vi "Master Setup File Fault Check.vi"(0 "Reset?":bool, 5 "Clear File Load Error Ref.":refnum<vi>, 7 "Pattern Label":T2 items=["Channel Setup (0)", "PID Setup (1)", "Filter Setup (2)", "~Reserved Old CAN Msgs (3)", "~Reserved Old CAN1 (4)", "~Reserved Old CAN2 (5)", "Digital Inputs Setup (6)", "Digital Outputs Setup (7)", "Logging 1 Setup (8)", "Logging 2 Setup (9)", "Logging 3 Setup (10)", "Setpoint Setup (11)", "Test Series Setup (12)", "Graph Setup (13)", "System Configure (14)", "Header (15)", "Profile Manager (16)", "Post-Mortem Logging (17)", "High-Speed Data (18)", "Statistic Channel Setup (19)", "Ramp Channel Setup (20)", "ETAS INCA Channel Setup (21)", "ETC ECCS Transducer Setup (22)", "ETC ECCS Test Setup (23)", "AVL AK Smoke Meter Setup (24)", "Triggers Setup (25)", "Alarm Limits Setup (26)", "YKWT1 Measurement (27)", "YKWT1 Instrument (28)", "Auto File Settings (29)", "Playback File Setting (30)", "UUT Constants (31)", "UPS Setup (32)", "Differential Channel Setup (33)", "Integral Channel Setup (34)", "Signal Channel Setup (35)", "Calibration Setup (36)", "BNC Setup (37)", "ASAP3 Setup (38)", "Chassis Force Calculations (39)", "Chassis Teststand Losses (40)", "Chassis Vehicle Losses (41)", "Formula Channels (42)", "ASAP3 Map Coords Setup (43)", "Digital Controls Setup (44)", "Push Buttons Setup (45)", "Sliders Setup (46)", "~Reserved~ (47)", "Email Setup (48)", "Timer Setup (49)", "Unit Conversion Setup (50)", "Visible Channels (51)", "Main Display Setup (52)", "Message Display Setup (53)", "Input Display Setup (54)", "Unico Parameter Downloads (55)", "Flow Meter Setup (56)", "Channel Zero Offset (57)", "YKWT2 Measurement (58)", "YKWT2 Instrument (59)", "~Reserved Old CAN3 (60)", "CAS Setup (61)", "Accumulation Channel Setup (62)", "Valvetrain Dynamics Setup (63)", "CCP Setup (64)", "System Log Setup (65)", "Throttle Controller (66)", "RE Shifter (67)", "Main Display (68)", "~Reserved~ (69)", "FlexRay (70)", "YKWT3 Measurement (71)", "YKWT3 Instrument (72)", "CAN XNET API (73)"], 9 "File Operation":T1, 11 "error in (no error)":errorcluster) -> (4 "Module Fault Array":bool[](array[boolean]), 15 "error out":errorcluster)   [LabVIEW 2017]
uses:
  Master Setup Pattern Enum.ctl
  Setup File Operations/File Operation with History.ctl
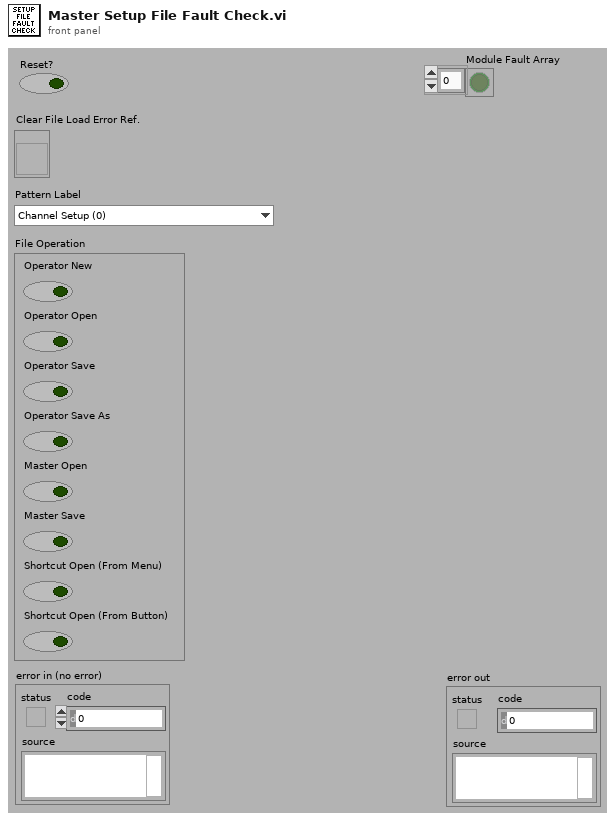
[diagram p1: front panel]
types:
  T1 = typedef "File Operation with History.ctl" = cluster{"Operator New":bool, "Operator Open":bool, "Operator Save":bool, "Operator Save As":bool, "Master Open":bool, "Master Save":bool, "Shortcut Open (From Menu)":bool, "Shortcut Open (From Button)":bool}
  T2 = typedef "Master Setup Pattern Enum.ctl" = i32
  T3 = typedef "PC_INI_Data__TypeDef.ctl" = cluster{"REPS Version":T4, "System Configuration":T5, "OPC PLC Write":string, "OPC PLC Read":string, "Modbus Info":string, "INCA Configuration":cluster{"IP":string, "Port":i32, "Protocol Version":i32}, "ECCS Setup":cluster{"Enable":bool, "IP":string, "TCP Port":u16, "UDP Port":u16, "Engine ODBC Name":string, "Fuel ODBC Name":string}, "Encoder Configuration":cluster{"Encoder1PPR":i32, "Encoder1Interval1":i32, "Encoder1Interval2":i32, "Roll Diameter(Feet)":i32, "Encoder2PPR":i32, "Encoder3PPR":i32, "Encoder4PPR":i32, "Encoder5PPR":i32, "Encoder2Interval1":i32, "Encoder2Interval2":i32, "Encoder3Interval1":i32, "Encoder3Interval2":i32}, "Pickup1 Configuration":cluster{"PickupPPR":i32, "PickupInterval1":i32, "PickupInterval2":i32}, "Pickup2 Configuration":cluster{"PickupPPR":i32, "PickupInterval1":i32, "PickupInterval2":i32}, "Pickup3 Configuration":cluster{"PickupPPR":i32, "PickupInterval1":i32, "PickupInterval2":i32}, "Shifter Configuration":cluster{"RE Shifter Enable":bool, "Shifter IP Address":string, "Shifter Port":u16}, "Misc Configuration":T6, "Logging Configuration":cluster{"Number of Log Channels":dbl, "Max Log  File Size":dbl}}
  T4 = typedef "REPS Version.ctl" = cluster{"Version":string}
  T5 = typedef "System Configuration.ctl" = cluster{"Cell":string, "DualMotorSet":bool, "Hardware Setup Array":bool[], "Host IP":string, "Remote IP 1":string, "Remote IP 2":string, "Remote IP 3":string, "Remote Enable 1":bool, "Remote Enable 2":bool, "Remote Enable 3":bool, "Company Name":string, "Company Info":string, "Number Of Modbus":i32, "Setup Files Path":path, "Master File Path":path, "Master Setup Titles":string[], "Encoder1PPR":i32, "Encoder1Interval1":i32, "Encoder1Interval2":i32, "Display File Error Status?":bool[], "Update to RT Delay":u32, "Formula Rate (Hz)":u32, "Custom Screen (Left) Path":path, "Custom Screen (Right) Path":path}
  T6 = typedef "Misc Configuration.ctl" = cluster{"Show PM Logging Indicator":bool}
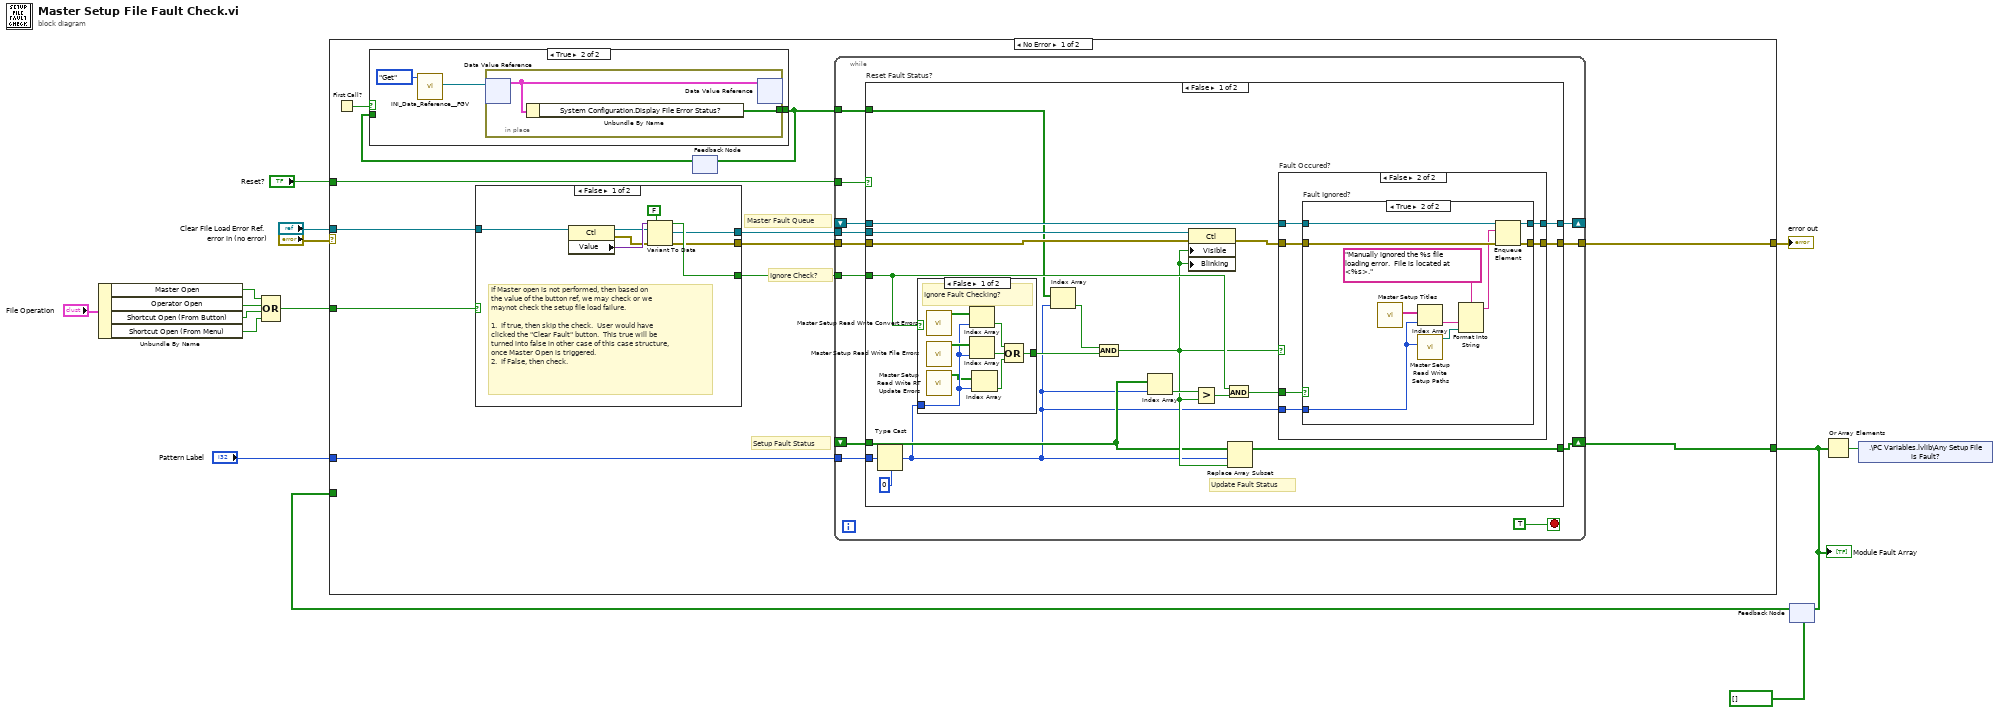
[diagram p0: block diagram]
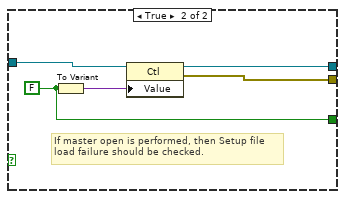
[diagram p3: hidden frame]
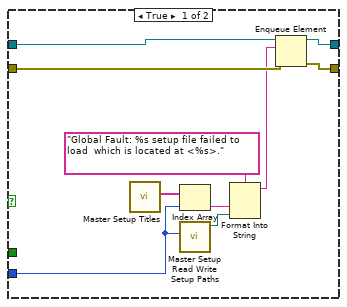
[diagram p4: hidden frame]
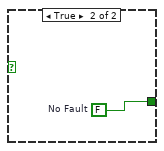
[diagram p6: hidden frame]
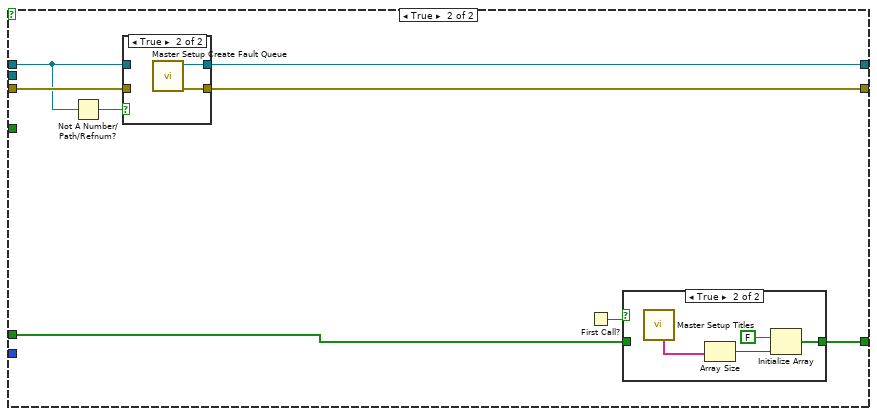
[diagram p7: hidden frame]
diagram:
  n1 = Unbundle By Name("File Operation") -> ("Master Open"=w10:bool, "Operator Open"=w12:bool, "Shortcut Open (From Button)"=w13:bool, "Shortcut Open (From Menu)"=w14:bool)
  n2 = Compound Arithmetic op=OR(w10, w12, w13, w14) -> (w11:bool)
  n3 = feedback #1(bool[] []) -> (w1:bool[])
  n4 = case shown="No Error" "error in (no error)" {
    selector: "error in (no error)" -> [_ w132]
    tunnel: [w27 w132] -> w15
    tunnel: w11 -> [w26 _]
    tunnel: "Clear File Load Error Ref." -> [w23 _]
    tunnel: "Pattern Label" -> [w21 _]
    tunnel: "Reset?" -> [w20 _]
    tunnel: [w19 w131] -> w3
    tunnel: w1 -> [_ w131]
    frame No Error {
      # "Master Fault Queue"
      # "Ignore Check?"
      # "Setup Fault Status"
      n5 = First Call?() -> (First Call?: T/F=w18:bool)
      n6 = case shown="False" w26 {
        tunnel: [w37 w44] -> w25
        tunnel: [w36 w43] -> w24
        tunnel: w23 -> [w35 w42]
        tunnel: [w34 w41] -> w22
        frame False {
          # "If Master open is not performed, then based on\nthe value of the button ref, we may check or we\nmaynot check the setup file load failure.\n\n1.  If true, then skip the check.  User would have\nclicked the \"Clear Fault\" button.  This true will be\nturned into false in other case of this case structure,\nonce Master Open is triggered.\n2.  If False, then check."
          n7 = property class="Ctl"(reference=w35) -> (reference out=w34:refnum<vi>, error out=w38:errorcluster, "Value"=w39:variant)  [unwired: 1 in]
          n8 = Variant To Data(error in=w38, type=FALSE, Variant=w39) -> (data=w37:bool, error out=w36:errorcluster)
        }
        frame True {
          w44 = FALSE
          # "If master open is performed, then Setup file\nload failure should be checked."
          n9 = To Variant(anything=w44) -> (Variant=w45:variant)
          n10 = property class="Ctl"(reference=w42, "Value"=w45) -> (reference out=w41:refnum<vi>, error out=w43:errorcluster)  [unwired: 1 in]
        }
      }
      n11 = feedback #2() -> (w17:bool[])  [unwired: 1 in]
      n12 = case shown="True" w18 {
        tunnel: [w28 w30] -> w16
        tunnel: w17 -> [w28 _]
        frame False {
        }
        frame True {
          n13 = call "INI_Data_Reference__FGV.vi"("Action (Get)"=enum16{"Get", "Set"}."Get") -> (".ini Data Value Reference (out)"=w29:refnum<data-value>)  [unwired: 10 in]
          n14 = in-place {
            in-place-border: [w33] -> w30
            n15 = in-place-dvr #3(w29) -> (w32:T3)  [unwired: 1 out]
            n16 = Unbundle By Name(w32) -> ("System Configuration.Display File Error Status?"=w33:bool[])
            n17 = in-place-dvr #3(w32) -> ()  [unwired: 2 out]
          }
        }
      }
      n18 = feedback-in #2(w16) -> ()
      n19 = while {
        tunnel: w21 -> [w55]
        shift-right: [w56] -> w19
        shift-left: _ -> [w51]
        tunnel: w20 -> [w52]
        tunnel: w25 -> [w54]
        tunnel: w22 -> [w53]
        tunnel: [w50] -> w27
        tunnel: w24 -> [w49]
        shift-right: [w48] -> _
        shift-left: _ -> [w47]
        tunnel: w16 -> [w46]
        stop <- TRUE stop-if-true
        n20 = case "Reset Fault Status?" shown="False" w52 {
          tunnel: w51 -> [w60 w115]
          tunnel: [w76 w121] -> w56
          tunnel: w55 -> [w65 _]
          tunnel: w54 -> [w64 _]
          tunnel: w53 -> [w75 _]
          tunnel: [w70 w119] -> w50
          tunnel: w49 -> [w74 w118]
          tunnel: [w73 w120] -> w48
          tunnel: w47 -> [w72 w117]
          tunnel: w46 -> [w61 _]
          frame False {
            # "Update Fault Status"
            n21 = Type Cast(type=0 ("index"), x=w65) -> (*(type *) &x=w59:i32)
            n22 = case shown="False" w64 {
              tunnel: w59 -> [w106 _]
              tunnel: [w107 w113] -> w63
              frame False {
                # "Ignore Fault Checking?"
                n23 = call "Master Setup Read Write Convert Errors.vi"() -> ("Convert Error (out)"=w111:bool[])  [unwired: 10 in, 1 out]
                n24 = call "Master Setup Read Write File Errors.vi"() -> ("File Error (out)"=w112:bool[])  [unwired: 10 in, 1 out]
                n25 = call "Master Setup Read Write RT Update Errors.vi"() -> ("Real-Time Update Status (out)"=w105:bool[])  [unwired: 9 in, 2 out]
                n26 = Index Array(array=w111, index=w106) -> (element=w110:bool)
                n27 = Index Array(array=w112, index=w106) -> (element=w109:bool)
                n28 = Index Array(array=w105, index=w106) -> (element=w108:bool)
                n29 = Compound Arithmetic op=OR(w110, w109, w108) -> (w107:bool)
              }
              frame True {
                w113 = FALSE  # No Fault
              }
            }
            n30 = Index Array(array=w61, index=w59) -> (element=w58:bool)
            n31 = And(x=w58, y=w63) -> (x .and. y?=w62:bool)
            n32 = Index Array(array=w60, index=w59) -> (element=w69:bool)
            n33 = property class="Ctl"(reference=w75, error in=w74, "Visible"=w62, "Blinking"=w62) -> (error out=w71:errorcluster)  [unwired: 1 out]
            n34 = Greater?(x=w69, y=w62) -> (0:w68:bool)
            n35 = And(x=w64, y=w68) -> (x .and. y?=w67:bool)
            n36 = Replace Array Subset(array=w60, new element=w62, index=w59) -> (w76:bool[])
            n37 = case "Fault Occured?" shown="False" w62 {
              tunnel: w72 -> [w86 w92]
              tunnel: [w85 w91] -> w73
              tunnel: w71 -> [w84 w90]
              tunnel: [w83 w89] -> w70
              tunnel: w59 -> [w81 w88]
              tunnel: w67 -> [_ w87]
              frame True {
                n38 = call "Master Setup Titles.vi"() -> ("Setup Description"=w82:string[])  [unwired: 6 in, 5 out]
                n39 = Index Array(array=w82, index=w81) -> (element=w79:string)
                n40 = call "Master Setup Read Write Setup Paths.vi"("Pattern Label"=w81) -> ("New Setup Path"=w78:path)  [unwired: 6 in, 4 out]
                n41 = Format Into String(format string="Global Fault: %s setup file failed to load  which is located at <%s>." ("[Date/Time] [Fault Status] [Fault Type] ... [Channel Name] ... [Value] ... [Limit]"), w79, w78) -> (resulting string=w77:string)  [unwired: 2 in, 1 out]
                n42 = Enqueue Element(queue=w86, element=w77, error in (no error)=w84) -> (queue out=w85:refnum<queue>, error out=w83:errorcluster)  [unwired: 1 in, 1 out]
              }
              frame False {
                n43 = case "Fault Ignored?" shown="True" w87 {
                  tunnel: w92 -> [w94 w104]
                  tunnel: [w94 w103] -> w91
                  tunnel: w90 -> [w93 w102]
                  tunnel: [w93 w101] -> w89
                  tunnel: w88 -> [_ w99]
                  frame False {
                  }
                  frame True {
                    n44 = call "Master Setup Titles.vi"() -> ("Setup Description"=w100:string[])  [unwired: 6 in, 5 out]
                    n45 = Index Array(array=w100, index=w99) -> (element=w97:string)
                    n46 = call "Master Setup Read Write Setup Paths.vi"("Pattern Label"=w99) -> ("New Setup Path"=w96:path)  [unwired: 6 in, 4 out]
                    n47 = Format Into String(format string="Manually ignored the %s file loading error.  File is located at <%s>." ("[Date/Time] [Fault Status] [Fault Type] ... [Channel Name] ... [Value] ... [Limit]"), w97, w96) -> (resulting string=w95:string)  [unwired: 2 in, 1 out]
                    n48 = Enqueue Element(queue=w104, element=w95, error in (no error)=w102) -> (queue out=w103:refnum<queue>, error out=w101:errorcluster)  [unwired: 1 in, 1 out]
                  }
                }
              }
            }
          }
          frame True {
            n49 = Not A Number/Path/Refnum?(number/path/refnum=w117) -> (NaN/Path/Refnum?=w116:bool)
            n50 = case shown="True" w116 {
              tunnel: [w128 w130] -> w120
              tunnel: w117 -> [w128 _]
              tunnel: [w127 w129] -> w119
              tunnel: w118 -> [w127 _]
              frame False {
              }
              frame True {
                n51 = call "Master Setup Create Fault Queue.vi"() -> ("error out"=w129:errorcluster, "Master Fault Queue"=w130:refnum<queue>)  [unwired: 6 in]
              }
            }
            n52 = First Call?() -> (First Call?: T/F=w114:bool)
            n53 = case shown="True" w114 {
              tunnel: [w122 w126] -> w121
              tunnel: w115 -> [w122 _]
              frame False {
              }
              frame True {
                n54 = call "Master Setup Titles.vi"() -> ("Sorted Setup Description"=w124:string[])  [unwired: 6 in, 5 out]
                n55 = Array Size(array=w124) -> (size(s)=w123:i32)
                n56 = Initialize Array(FALSE ("Reset?"), w123) -> (w126:bool[])
              }
            }
          }
        }
      }
    }
    frame Error {
    }
  }
  "error out" <- w15
  "Module Fault Array" <- w3
  n57 = feedback-in #1(w3) -> ()
  n58 = Or Array Elements(Boolean array=w3) -> (logical OR=w4:bool)
  n59 = shared-variable ".\\PC Variables.lvlib\\Any Setup File is Fault?"(w4) -> ()  [unwired: 1 in, 1 out]
